vi "IMU Functions.vi"() -> ()   [LabVIEW 2026]
uses:
  <menus>/Categories/MRC/MrcLib.lvlib
  vi.lib/MRC/MrcLib/VIs/IMU/IMU Get Euler Angle Flat.vi
  vi.lib/MRC/MrcLib/VIs/IMU/IMU Get Yaw Flat.vi
  vi.lib/MRC/Types/MRC 3D Acceleration Values.ctl
  vi.lib/MRC/Types/MRC Euler Angles Values.ctl
  vi.lib/MRC/Types/MRC Gyro Rates Values.ctl
  vi.lib/MRC/Types/MRC Quaternion Values.ctl
panel:
  out "quaternion":T1
  out "rates":T2
  out "Euler angles":T3
  out "acceleration":T4
  out "yaw out":dbl
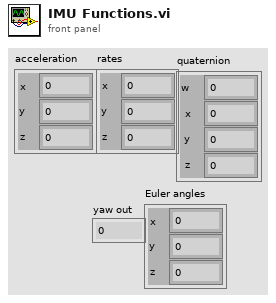
[diagram p1: front panel]
types:
  T1 = typedef "MrcLib.lvlib/MRC Quaternion Values.ctl" = cluster{"w":dbl, "x":dbl, "y":dbl, "z":dbl}
  T2 = typedef "MrcLib.lvlib/MRC Gyro Rates Values.ctl" = cluster{"x":dbl, "y":dbl, "z":dbl}
  T3 = typedef "MrcLib.lvlib/MRC Euler Angles Values.ctl" = cluster{"x":dbl, "y":dbl, "z":dbl}
  T4 = typedef "MrcLib.lvlib/MRC 3D Acceleration Values.ctl" = cluster{"x":dbl, "y":dbl, "z":dbl}
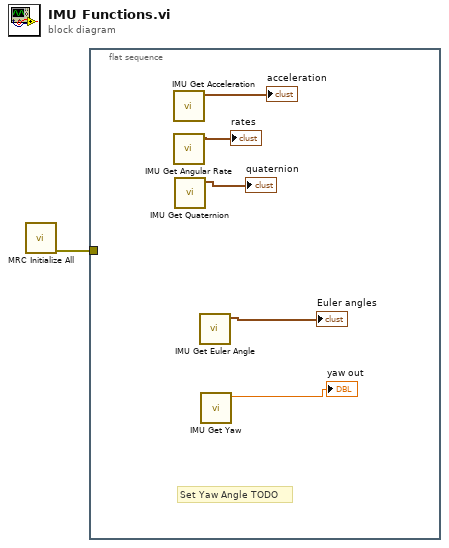
[diagram p0: block diagram]
diagram:
  n1 = call "MRC Initialize All.vi"() -> ("error out"=w1:errorcluster)  [unwired: 11 in]
  n2 = flat-sequence {
    tunnel: w1 -> [_]
    frame #0 {
      # "Set Yaw Angle TODO"
      n3 = call "IMU Get Acceleration.vi"() -> ("acceleration"=→"acceleration":T4)  [unwired: 9 in, 2 out]
      n4 = call "IMU Get Angular Rate.vi"() -> ("rates"=→"rates":T2)  [unwired: 9 in, 2 out]
      n5 = call "IMU Get Quaternion.vi"() -> ("quaternion"=→"quaternion":T1)  [unwired: 9 in, 2 out]
      n6 = call-poly "IMU Get Euler Angle.vi"() -> ("Euler angles"=→"Euler angles":T3)  [unwired: 9 in, 2 out]
      n7 = call-poly "IMU Get Yaw.vi"() -> ("yaw out"=→"yaw out":dbl)  [unwired: 9 in, 2 out]
    }
  }
